vi "Databse State Checker Testing.vi"(8 "error in":errorcluster, 9 "connection information":path, 10 "System Number":string, 11 "Arduino":refnum<visa-resource-name>="COM4") -> (0 "error out":errorcluster, 3 "Arduino out":refnum<visa-resource-name>)   [LabVIEW 2024]
uses:
  <vilib>/addons/database/Connection.llb/DB Tools Open Connec (Path).vi
  <vilib>/addons/database/_DB Variant To Data/Database Variant To Data.xnode
  <vilib>/regexp/Match Regular Expression.xnode
  <vilib>/addons/database/NI_Database_API.lvlib
panel:
  out "Command Array":string[](array[string])
  in  "Database Available?":bool=TRUE
  out "Power":string[](array[string])
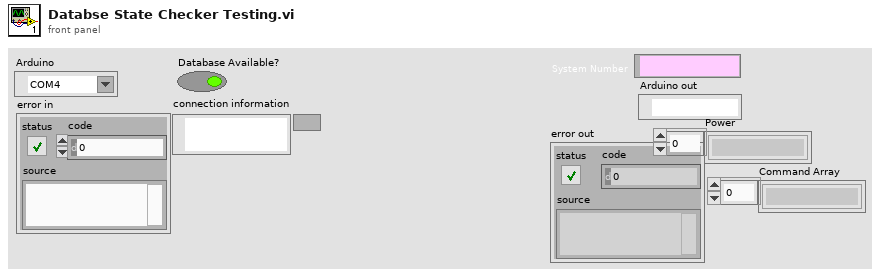
[diagram p1: front panel]
types:
  T1 = typedef "NI_Database_API.lvlib/Conn ObjectReference.ctl" = refnum<k1>
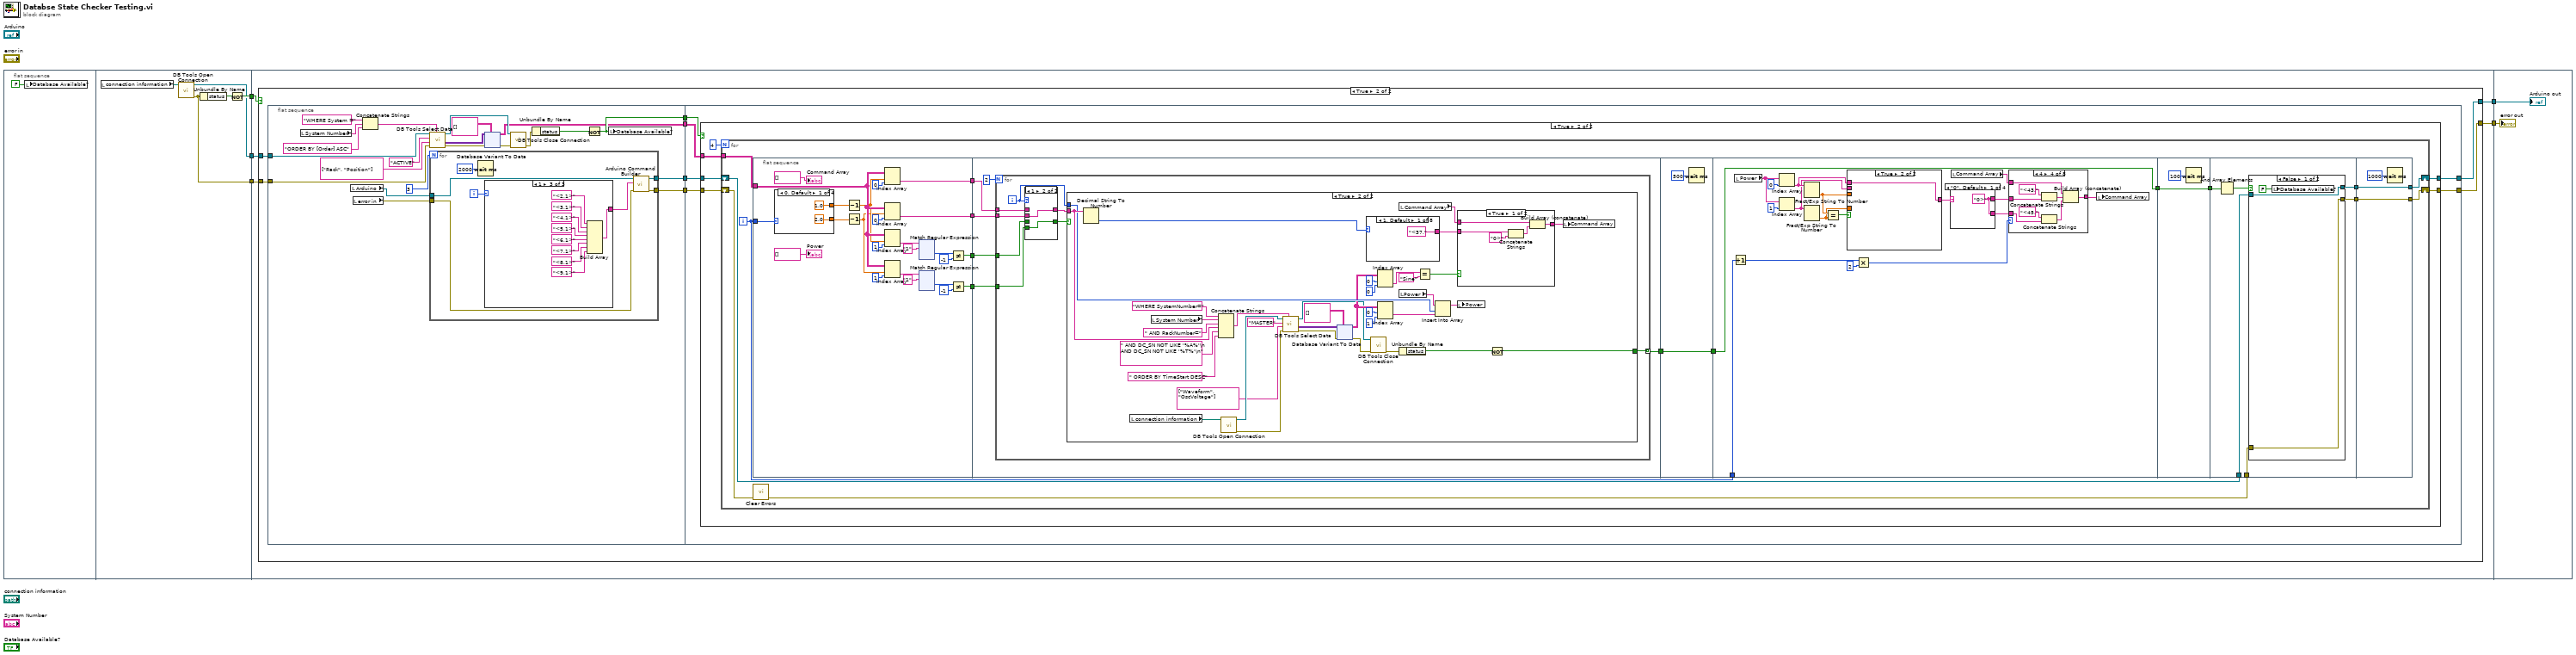
[diagram p0: block diagram]
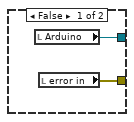
[diagram p2: hidden frame]
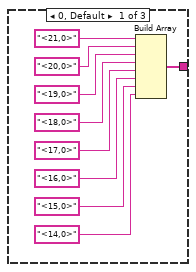
[diagram p3: hidden frame]
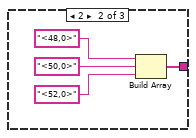
[diagram p4: hidden frame]
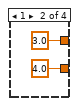
[diagram p6: hidden frame]
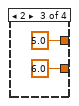
[diagram p7: hidden frame]
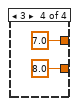
[diagram p8: hidden frame]
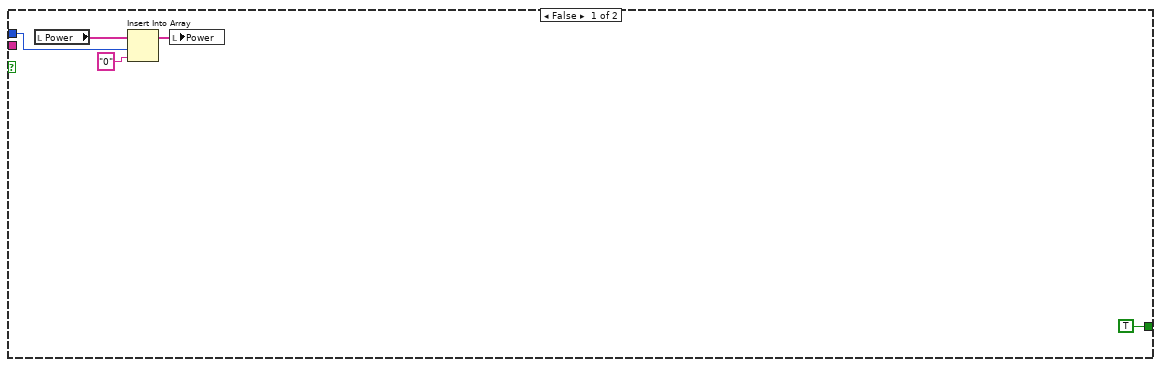
[diagram p10: hidden frame]
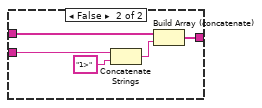
[diagram p11: hidden frame]
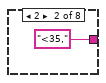
[diagram p12: hidden frame]
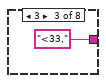
[diagram p13: hidden frame]
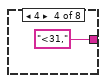
[diagram p14: hidden frame]
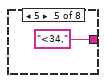
[diagram p15: hidden frame]
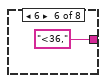
[diagram p16: hidden frame]
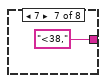
[diagram p17: hidden frame]
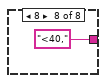
[diagram p18: hidden frame]
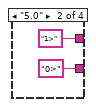
[diagram p19: hidden frame]
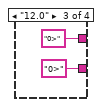
[diagram p20: hidden frame]
diagram:
  n1 = flat-sequence {
    tunnel: [w9] -> w3
    tunnel: [w8] -> w2
    tunnel: [w10] -> w1
    tunnel: [w15] -> w5
    tunnel: [w16] -> w4
    tunnel: w3 -> [w13]
    tunnel: w2 -> [w12]
    tunnel: w1 -> [w14]
    tunnel: w5 -> [w660]
    tunnel: w4 -> [w659]
    frame #0 {
      n2 = local write "Database Available?"(FALSE ("Database Available?")) -> ()
    }
    frame #1 {
      n3 = local read "connection information"() -> (w7:path)
      n4 = call-poly <vilib>:"DB Tools Open Connection.vi"("connection information"=w7) -> ("error out"=w8:errorcluster, "connection reference"=w9:T1)  [unwired: 7 in]
      n5 = Unbundle By Name(w8) -> ("status"=w11:bool)
      n6 = Not(x=w11) -> (.not. x?=w10:bool)
    }
    frame #2 {
      n7 = case shown="True" w14 {
        tunnel: [w18 w22] -> w16
        tunnel: [w17 w21] -> w15
        tunnel: w13 -> [_ w20]
        tunnel: w12 -> [_ w19]
        frame False {
          n8 = local read "Arduino"() -> (w18:refnum<visa-resource-name>)
          n9 = local read "error in"() -> (w17:errorcluster)
        }
        frame True {
          n10 = flat-sequence {
            tunnel: w20 -> [w32]
            tunnel: w19 -> [w31]
            tunnel: [w40] -> w26
            tunnel: [w41] -> w25
            tunnel: [w33] -> w24
            tunnel: [w44] -> w23
            tunnel: [w127] -> w22
            tunnel: [w126] -> w21
            tunnel: w26 -> [w123]
            tunnel: w25 -> [w122]
            tunnel: w24 -> [w125]
            tunnel: w23 -> [w124]
            frame #0 {
              n11 = local read "System Number"() -> (w48:string)
              n12 = local read "Arduino"() -> (w42:refnum<visa-resource-name>)
              n13 = local read "error in"() -> (w43:errorcluster)
              n14 = Concatenate Strings("WHERE System =" ("ConnectionString In"), w48, "ORDER BY [Order] ASC" ("ConnectionString In")) -> (w28:string)
              n15 = call <vilib>:"DB Tools Select Data.vi"("condition"=w28, "error in (no error)"=w31, "columns"=string[] ["Rack", "Position"], "table"="ACTIVE", "connection reference"=w32) -> ("error out"=w38:errorcluster, "data"=w35:variant[][], "connection reference out"=w36:T1)  [unwired: 1 in]
              n16 = for {
                N: 3 -> [_]
                tunnel: w43 -> [w99]
                tunnel: w42 -> [w98]
                tunnel: [w97] -> w41
                tunnel: [w96] -> w40
                i -> [w95]
                n17 = Wait (ms)(milliseconds to wait=u32 2000) -> ()  [unwired: 1 out]
                n18 = case shown="1" w95 {
                  tunnel: [w100 w109 w113] -> w94
                  frame 0, Default {
                    n19 = Build Array("<21,0>" ("string"), "<20,0>" ("string"), "<19,0>" ("string"), "<18,0>" ("string"), "<17,0>" ("string"), "<16,0>" ("string"), "<15,0>" ("string"), "<14,0>" ("string")) -> (w100:string[])
                  }
                  frame 2 {
                    n20 = Build Array("<48,0>" ("string"), "<50,0>" ("string"), "<52,0>" ("string")) -> (w109:string[])
                  }
                  frame 1 {
                    n21 = Build Array("<2,1>" ("string"), "<3,1>" ("string"), "<4,1>" ("string"), "<5,1>" ("string"), "<6,1>" ("string"), "<7,1>" ("string"), "<8,1>" ("string"), "<9,1>" ("string")) -> (w113:string[])
                  }
                }
                n22 = call "Arduino Command Builder.vi"("error in"=w99, "Commands"=w94, "Arduino in"=w98) -> ("error out"=w97:errorcluster, "Arduino out"=w96:refnum<visa-resource-name>)  [unwired: 7 in]
              }
              n23 = xnode "Database Variant To Data"("database variant"=w35, "error in (no error)"=w38, "type"=string[][] [] ("Power")) -> ("data"=w33:string[][], "error out"=w37:errorcluster)
              n24 = call <vilib>:"DB Tools Close Connection.vi"("error in (no error)"=w37, "connection reference"=w36) -> ("error out"=w30:errorcluster)  [unwired: 5 in]
              n25 = Unbundle By Name(w30) -> ("status"=w45:bool)
              n26 = Not(x=w45) -> (.not. x?=w44:bool)
              n27 = local write "Database Available?"(w44) -> ()
            }
            frame #1 {
              n28 = case shown="True" w124 {
                tunnel: [w129 w134] -> w127
                tunnel: [w128 w133] -> w126
                tunnel: w125 -> [_ w132]
                tunnel: w123 -> [w129 w131]
                tunnel: w122 -> [w128 w130]
                frame False {
                }
                frame True {
                  n29 = for {
                    N: 4 -> [_]
                    tunnel: w132 -> [w152]
                    shift-right: [w150] -> w134
                    shift-left: w131 -> [w139]
                    shift-right: [w149] -> w133
                    shift-left: w130 -> [w145]
                    i -> [w144]
                    n30 = flat-sequence {
                      tunnel: [w155] -> w151
                      tunnel: [w167] -> w148
                      tunnel: [w156] -> w147
                      tunnel: [w159] -> w146
                      tunnel: w144 -> [w166]
                      tunnel: w152 -> [w169]
                      tunnel: w151 -> [w424]
                      tunnel: w148 -> [w423]
                      tunnel: w147 -> [w422]
                      tunnel: w146 -> [w421]
                      tunnel: [w419] -> w140
                      tunnel: [w540] -> w141
                      tunnel: w140 -> [w540]
                      tunnel: w144 -> [w548]
                      tunnel: [w542] -> w142
                      tunnel: w141 -> [w542]
                      tunnel: [w640] -> w143
                      tunnel: w142 -> [w640]
                      tunnel: w143 -> [w647]
                      tunnel: w139 -> [w644]
                      tunnel: w138 -> [w645]
                      tunnel: [w643] -> w137
                      tunnel: [w642] -> w136
                      tunnel: [w657] -> w149
                      tunnel: [w658] -> w150
                      tunnel: w136 -> [w657]
                      tunnel: w137 -> [w658]
                      frame #0 {
                        n31 = case shown="0, Default" w166 {
                          tunnel: [1.0 3.0 5.0 7.0] -> w165
                          tunnel: [2.0 4.0 6.0 8.0] -> w164
                          frame 0, Default {
                          }
                          frame 1 {
                          }
                          frame 2 {
                          }
                          frame 3 {
                          }
                        }
                        n32 = Decrement(x=w165) -> (x-1=w163:dbl)
                        n33 = Decrement(x=w164) -> (x-1=w162:dbl)
                        n34 = Index Array(array=w169, index (row)=w163, index (col)=0 ("index")) -> (element=w159:string)
                        n35 = Index Array(array=w169, index (row)=w162, index (col)=0 ("index")) -> (element=w167:string)
                        n36 = Index Array(array=w169, index (row)=w163, index (col)=1 ("index")) -> (element=w158:string)
                        n37 = Index Array(array=w169, index (row)=w162, index (col)=1 ("index")) -> (element=w176:string)
                        n38 = xnode "Match Regular Expression"("input string"=w158, "regular expression"="1") -> ("offset past match"=w161:i32)  [unwired: 4 in, 4 out]
                        n39 = xnode "Match Regular Expression"("input string"=w176, "regular expression"="1") -> ("offset past match"=w175:i32)  [unwired: 4 in, 4 out]
                        n40 = Not Equal?(x=w161, y=-1) -> (x != y?=w156:bool)
                        n41 = Not Equal?(x=w175, y=-1) -> (x != y?=w155:bool)
                        "Power" <- string[] [] ("Power")
                        "Command Array" <- string[] [] ("Power")
                      }
                      frame #1 {
                        n42 = for {
                          N: 2 -> [_]
                          tunnel: w424 -> [w431]
                          tunnel: w423 -> [w428]
                          tunnel: w422 -> [w432]
                          tunnel: w421 -> [w429]
                          tunnel: [w425] -> w419 mode=indexing
                          i -> [w426]
                          n43 = case shown="1" w426 {
                            tunnel: w432 -> [w434 _]
                            tunnel: [w434 w436] -> w430
                            tunnel: w431 -> [_ w436]
                            tunnel: w429 -> [w433 _]
                            tunnel: w428 -> [_ w435]
                            tunnel: [w433 w435] -> w427
                            frame 0, Default {
                            }
                            frame 1 {
                            }
                          }
                          n44 = case shown="True" w430 {
                            tunnel: w427 -> [_ w477]
                            tunnel: w426 -> [w441 w476]
                            tunnel: [TRUE w455] -> w425
                            frame False {
                              n45 = local read "Power"() -> (w440:string[])
                              n46 = Insert Into Array(array=w440, index=w441, new element="0" ("new element/subarray")) -> (w439:string[])
                              n47 = local write "Power"(w439) -> ()
                            }
                            frame True {
                              n48 = Decimal String To Number(string=w477) -> (number=w466:i32)  [unwired: 2 in, 1 out]
                              n49 = local read "connection information"() -> (w442:path)
                              n50 = local read "System Number"() -> (w473:string)
                              n51 = Concatenate Strings("WHERE SystemNumber=" ("string"), w473, " AND RackNumber=", w477, " AND DC_SN NOT LIKE '%A%'\n  AND DC_SN NOT LIKE '%T%'\n" ("string"), " ORDER BY TimeStart DESC" ("string")) -> (w446:string)
                              n52 = call-poly <vilib>:"DB Tools Open Connection.vi"("connection information"=w442) -> ("error out"=w450:errorcluster, "connection reference"=w451:T1)  [unwired: 7 in]
                              n53 = call <vilib>:"DB Tools Select Data.vi"("condition"=w446, "error in (no error)"=w450, "columns"=string[] ["Waveform", "OscVoltage"], "table"="MASTER", "connection reference"=w451) -> ("error out"=w454:errorcluster, "data"=w452:variant[][], "connection reference out"=w443:T1)  [unwired: 1 in]
                              n54 = xnode "Database Variant To Data"("database variant"=w452, "error in (no error)"=w454, "type"=string[][] [] ("Power")) -> ("data"=w448:string[][], "error out"=w453:errorcluster)
                              n55 = case shown="1, Default" w466 {
                                tunnel: ["<37," ("y") "<35," ("y") "<33," ("y") "<31," ("y") "<34," ("y") "<36," ("y") "<38," ("y") "<40," ("y")] -> w460
                                frame 1, Default {
                                }
                                frame 2 {
                                }
                                frame 3 {
                                }
                                frame 4 {
                                }
                                frame 5 {
                                }
                                frame 6 {
                                }
                                frame 7 {
                                }
                                frame 8 {
                                }
                              }
                              n56 = call <vilib>:"DB Tools Close Connection.vi"("error in (no error)"=w453, "connection reference"=w443) -> ("error out"=w447:errorcluster)  [unwired: 5 in]
                              n57 = Index Array(array=w448, index (row)=0 ("index"), index (col)=0 ("disabled index (col)")) -> (element=w468:string)
                              n58 = Index Array(array=w448, index (row)=0, index (col)=1 ("disabled index (col)")) -> (element=w465:string)
                              n59 = local read "Power"() -> (w463:string[])
                              n60 = Unbundle By Name(w447) -> ("status"=w456:bool)
                              n61 = local read "Command Array"() -> (w459:string[])
                              n62 = Equal?(x=w468, y="Sine") -> (x = y?=w457:bool)
                              n63 = Insert Into Array(array=w463, index=w476, new element=w465) -> (w464:string[])
                              n64 = case shown="True" w457 {
                                tunnel: w460 -> [w525 w530]
                                tunnel: [w524 w529] -> w458
                                tunnel: w459 -> [w523 w528]
                                frame True {
                                n65 = Concatenate Strings(w525, "0>" ("y")) -> (w522:string)
                                n66 = Build Array (concatenate)(w523, w522) -> (w524:string[])
                                }
                                frame False {
                                n67 = Concatenate Strings(w530, "1>" ("y")) -> (w527:string)
                                n68 = Build Array (concatenate)(w528, w527) -> (w529:string[])
                                }
                              }
                              n69 = local write "Power"(w464) -> ()
                              n70 = Not(x=w456) -> (.not. x?=w455:bool)
                              n71 = local write "Command Array"(w458) -> ()
                            }
                          }
                        }
                      }
                      frame #2 {
                        n72 = Wait (ms)(milliseconds to wait=u32 500) -> ()  [unwired: 1 out]
                      }
                      frame #3 {
                        n73 = Increment(x=w548) -> (x+1=w549:i32)
                        n74 = local read "Power"() -> (w557:string[])
                        n75 = Index Array(array=w557, index=0) -> (element=w553:string)
                        n76 = Index Array(array=w557, index=1) -> (element=w552:string)
                        n77 = Fract/Exp String To Number(string=w553) -> (number=w551:dbl)  [unwired: 3 in, 1 out]
                        n78 = Fract/Exp String To Number(string=w552) -> (number=w550:dbl)  [unwired: 3 in, 1 out]
                        n79 = Equal?(x=w551, y=w550) -> (x = y?=w554:bool)
                        n80 = case shown="True" w554 {
                          tunnel: w553 -> [w569 w575]
                          tunnel: [w567 w575] -> w545
                          tunnel: w552 -> [w568 _]
                          tunnel: w551 -> [w572 _]
                          tunnel: w550 -> [w571 _]
                          frame False {
                            n81 = Greater?(x=w572, y=w571) -> (0:w570:bool)
                            n82 = case shown="True" w570 {
                              tunnel: w569 -> [_ w574]
                              tunnel: w568 -> [w573 _]
                              tunnel: [w573 w574] -> w567
                              frame False {
                              }
                              frame True {
                              }
                            }
                          }
                          frame True {
                          }
                        }
                        n83 = Multiply(x=w549, y=2) -> (x*y=w546:i32)
                        n84 = case shown="\"0\", Default" w545 {
                          tunnel: [w560 "1>" ("y") "0>" ("y") "0>" ("y")] -> w544
                          tunnel: [w560 "0>" ("y") "0>" ("y") "0>" ("y")] -> w543
                          frame "0", Default {
                            w560 = "0>" ("y")
                          }
                          frame "5.0" {
                          }
                          frame "12.0" {
                          }
                          frame "3.3" {
                          }
                        }
                        n85 = local read "Command Array"() -> (w559:string[])
                        n86 = case shown="4" w546 {
                          tunnel: w559 -> [w579 w587 w595 w603 w611 w619 w627 w635]
                          tunnel: [w578 w586 w594 w602 w610 w618 w626 w634] -> w558
                          tunnel: w544 -> [w581 w589 w597 w605 w613 w621 w629 w637]
                          tunnel: w543 -> [w580 w588 w596 w604 w612 w620 w628 w636]
                          frame 1, Default {
                            n87 = Concatenate Strings("<39," ("y"), w581) -> (w577:string)
                            n88 = Concatenate Strings("<41," ("y"), w580) -> (w576:string)
                            n89 = Build Array (concatenate)(w579, w577, w576) -> (w578:string[])
                          }
                          frame 2 {
                            n90 = Concatenate Strings("<39," ("y"), w589) -> (w585:string)
                            n91 = Concatenate Strings("<41," ("y"), w588) -> (w584:string)
                            n92 = Build Array (concatenate)(w587, w585, w584) -> (w586:string[])
                          }
                          frame 3 {
                            n93 = Concatenate Strings("<43," ("y"), w597) -> (w593:string)
                            n94 = Concatenate Strings("<45," ("y"), w596) -> (w592:string)
                            n95 = Build Array (concatenate)(w595, w593, w592) -> (w594:string[])
                          }
                          frame 4 {
                            n96 = Concatenate Strings("<43," ("y"), w605) -> (w601:string)
                            n97 = Concatenate Strings("<45," ("y"), w604) -> (w600:string)
                            n98 = Build Array (concatenate)(w603, w601, w600) -> (w602:string[])
                          }
                          frame 5 {
                            n99 = Concatenate Strings("<47," ("y"), w613) -> (w609:string)
                            n100 = Concatenate Strings("<49," ("y"), w612) -> (w608:string)
                            n101 = Build Array (concatenate)(w611, w609, w608) -> (w610:string[])
                          }
                          frame 6 {
                            n102 = Concatenate Strings("<47," ("y"), w621) -> (w617:string)
                            n103 = Concatenate Strings("<49," ("y"), w620) -> (w616:string)
                            n104 = Build Array (concatenate)(w619, w617, w616) -> (w618:string[])
                          }
                          frame 7 {
                            n105 = Concatenate Strings("<51," ("y"), w629) -> (w625:string)
                            n106 = Concatenate Strings("<53," ("y"), w628) -> (w624:string)
                            n107 = Build Array (concatenate)(w627, w625, w624) -> (w626:string[])
                          }
                          frame 8 {
                            n108 = Concatenate Strings("<51," ("y"), w637) -> (w633:string)
                            n109 = Concatenate Strings("<53," ("y"), w636) -> (w632:string)
                            n110 = Build Array (concatenate)(w635, w633, w632) -> (w634:string[])
                          }
                        }
                        n111 = local write "Command Array"(w558) -> ()
                      }
                      frame #4 {
                        n112 = Wait (ms)(milliseconds to wait=u32 100) -> ()  [unwired: 1 out]
                      }
                      frame #5 {
                        n113 = And Array Elements(Boolean array=w647) -> (logical AND=w646:bool)
                        n114 = case shown="False" w646 {
                          tunnel: w645 -> [w650 w655]
                          tunnel: w644 -> [w649 w654]
                          tunnel: [w649 w653] -> w643
                          tunnel: [w650 w652] -> w642
                          frame False {
                            n115 = local write "Database Available?"(FALSE ("Database Available?")) -> ()
                          }
                          frame True {
                            n116 = local read "Command Array"() -> (w651:string[])
                            n117 = call "Arduino Command Builder.vi"("error in"=w655, "Commands"=w651, "Arduino in"=w654) -> ("error out"=w652:errorcluster, "Arduino out"=w653:refnum<visa-resource-name>)  [unwired: 7 in]
                          }
                        }
                      }
                      frame #6 {
                        n118 = Wait (ms)(milliseconds to wait=u32 1000) -> ()  [unwired: 1 out]
                      }
                    }
                    n119 = call <vilib>:"Clear Errors.vi"("error in (no error)"=w145) -> ("error out"=w138:errorcluster)  [unwired: 5 in, 1 out]
                  }
                }
              }
            }
          }
        }
      }
    }
    frame #3 {
      "Arduino out" <- w659
      "error out" <- w660
    }
  }
